vi "Set JSON Scalar.vi"(8 "error in (no error)":errorcluster, 9 "Set as a JSON string (F)":bool, 10 "LabVIEW Text":string, 11 "JSON Scalar in":refnum<class "JSON Scalar.lvclass">) -> (0 "error out":errorcluster, 3 "JSON Scalar out":refnum<class "JSON Scalar.lvclass">)   [LabVIEW 2020, in "Library Commun.lvlib" / "JSON Scalar.lvclass"]
doc: "Stores a <b>String</b> as a <b>JSON Scalar</b>.\nUse <b>Set as a JSON string</b> to indicate it's a formatted string.\n\nCopyright 2012 James David Powell, Shaun Rumbell and Ton Plomp\nMore information on http://lavag.org/topic/16217-cr-json-labview"
uses:
  JSON Scalar.lvclass
  JSON Scalar.lvclass/JSON Scalar.ctl
  support/JSON support.lvlib
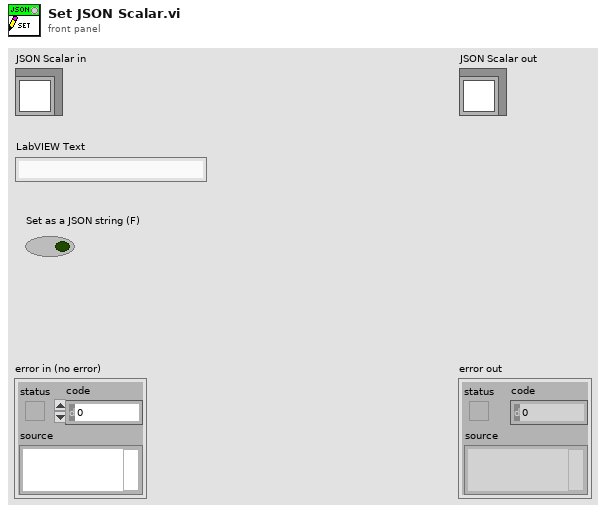
[diagram p1: front panel]
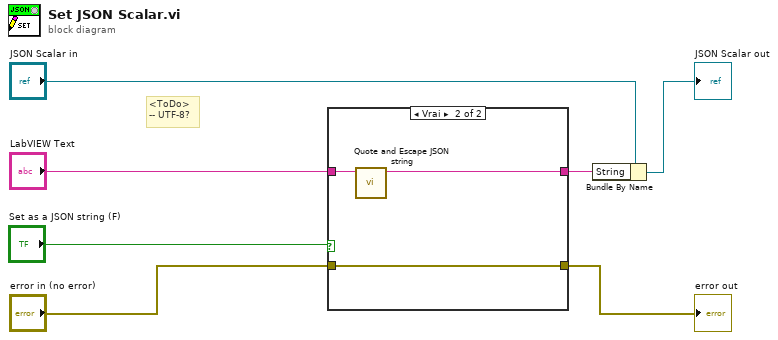
[diagram p0: block diagram]
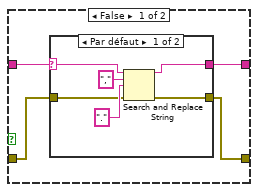
[diagram p2: hidden frame]
diagram:
  # "<ToDo>\n-- UTF-8?"
  n1 = case shown="Vrai" "Set as a JSON string (F)" {
    tunnel: [w10 w21] -> w1
    tunnel: "LabVIEW Text" -> [w11 w22]
    tunnel: "error in (no error)" -> [w9 w20]
    tunnel: [w8 w20] -> w6
    frame False {
      n2 = case shown="Par défaut" w11 {
        selector: w11 -> [w15 w19]
        tunnel: [w14 w19] -> w10
        tunnel: w9 -> [w13 w18]
        tunnel: [w12 w18] -> w8
        frame Default {
          n3 = Search and Replace String(input string=w15, search string=",", replace string="." ("replace string (\"\")"), error in=w13) -> (result string=w14:string, error out=w12:errorcluster)  [unwired: 4 in, 2 out]
        }
        frame "NaN" {
          # "<ToDo>"
        }
      }
    }
    frame True {
      n4 = call "Quote and Escape JSON string.vi"("Plain Text"=w22) -> ("<JSON>"=w21:string)  [unwired: 10 in]
    }
  }
  "error out" <- w6
  n5 = Bundle By Name(cluster="JSON Scalar in", "String"=w1) -> (→"JSON Scalar out":refnum<class "JSON Scalar.lvclass">)
